vi "Test Broadcast Latest Message ID Correct.vi"(8 "error in (no error)":errorcluster, 11 "Test Case In":refnum<class "Debugger Test.lvclass">) -> (0 "error out":errorcluster, 3 "Test Case Out":refnum<class "Debugger Test.lvclass">)   [LabVIEW 2020, in "Debugger Test.lvclass"]
uses:
  Debugger Test.lvclass
  Debugger Test.lvclass/Debugger Test.ctl
  source/Process/Debug Process.lvclass
  source/Debugger/Debugger.lvclass
  source/Debug Data/Debug Data.lvclass
  source/Debug Data/Raw Debug Data.ctl
  C:/Users/anton/Documents/GitHub/triarc-debugger/source/Process/Debug Process.lvclass
  C:/Users/anton/Documents/GitHub/triarc-debugger/source/Debugger/Debugger.lvclass
  C:/Users/anton/Documents/GitHub/triarc-debugger/source/Debug Data Event/Debug Data Listener.lvclass
  25a4e40d-e468-46ca-96f8-86723b982b85.vi
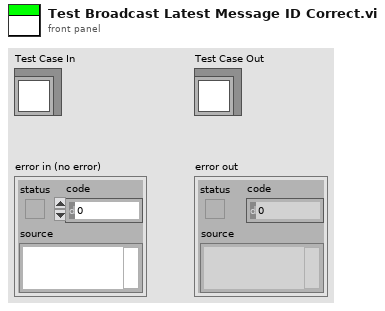
[diagram p1: front panel]
types:
  T1 = typedef "Debug Data.lvclass/Raw Debug Data.ctl" = cluster{"Action":string, "Call Chain":string, "Process":string, "Message":string, "Message Data":variant, "Time":dbl}
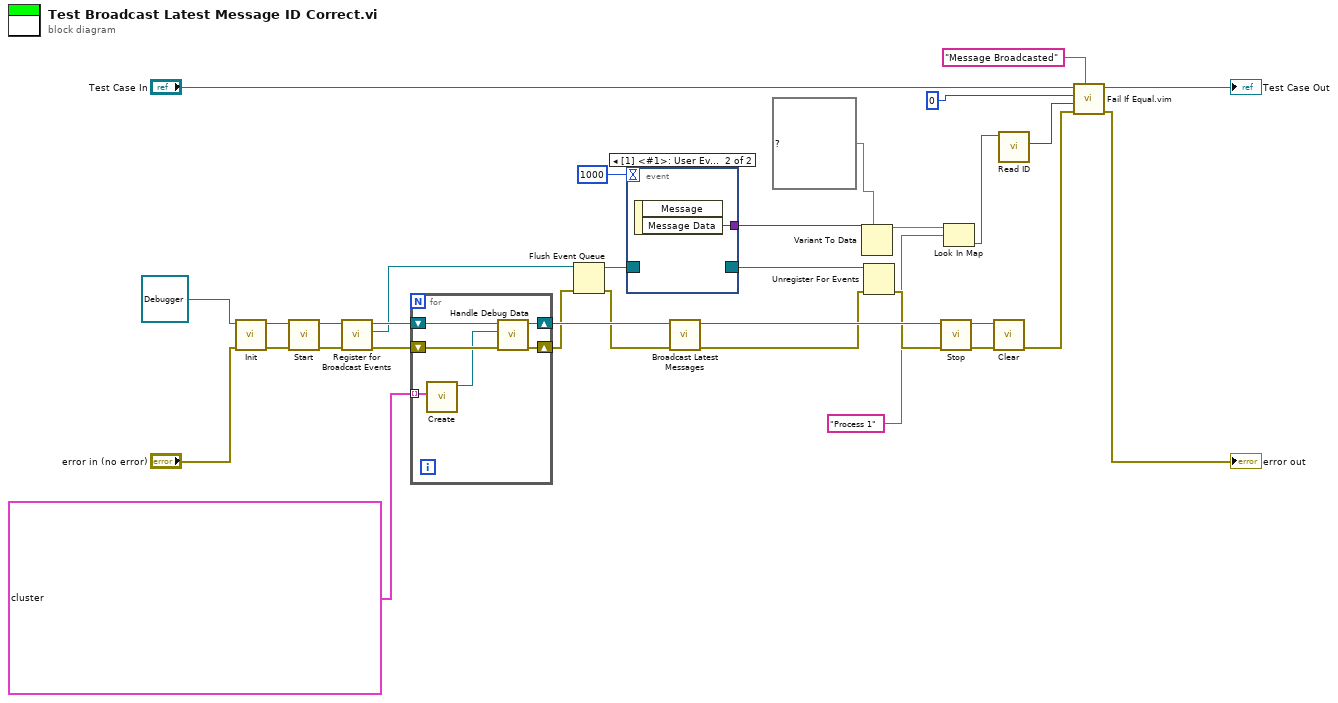
[diagram p0: block diagram]
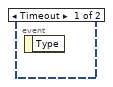
[diagram p2: hidden frame]
diagram:
  n1 = call-dynamic "Init.vi"("error in (no error)"="error in (no error)", "Process In"=refnum<class "Debugger.lvclass"> refnum ("Debug Data Event In 2")) -> ("error out"=w29:errorcluster, "Process Out"=w30:refnum<class "Debugger.lvclass">)  [unwired: 8 in]
  n2 = call "Start.vi"("error in (no error)"=w29, "Process In"=w30) -> ("error out"=w27:errorcluster, "Process Out"=w28:refnum<class "Debugger.lvclass">)  [unwired: 7 in, 1 out]
  n3 = call "Register for Broadcast Events.vi"("error in (no error)"=w27, "Process In"=w28) -> ("error out"=w26:errorcluster, "Event Registration Refnum Out"=w12:refnum<event-registration>, "Process Out"=w20:refnum<class "Debugger.lvclass">)  [unwired: 7 in]
  n4 = for {
    shift-right: [w37] -> w24
    shift-left: w26 -> [w39]
    shift-right: [w38] -> w25
    shift-left: w20 -> [w36]
    tunnel: T1[] [{"Action"="Send", "Call Chain"="Test.vi:123456", "Process"="Process 1", "Message"="Init", "Message Data"=variant, "Time"=0.0}, {"Action"="Receive", "Call Chain"="TF.lvlib:Process.lvclass:Handle Messages.vi:1960001", "Process"="Process 1", "Message"="Init", "Message Data"=variant, "Time"=0.0}, {"Action"="Send", "Call Chain"="Test.vi", "Process"="Process 1", "Message"="Start", "Message Data"=variant, "Time"=0.0}] ("Debug Data Cluster") -> [w35] mode=indexing
    n5 = call "Create.vi"("Debug Data Cluster"=w35) -> ("Debug Data out"=w34:refnum<class "Debug Data.lvclass">)  [unwired: 9 in, 1 out]
    n6 = call-dynamic "Handle Debug Data.vi"("error in (no error)"=w39, "Debug Data.lvclass"=w34, "Debug Data Event In"=w36) -> ("error out"=w37:errorcluster, "Debug Data Event Out"=w38:refnum<class "Debugger.lvclass">)  [unwired: 7 in]
  }
  n7 = Flush Event Queue(0:w12, 3:w24) -> (8:w11:refnum<event-registration>, 11:w13:errorcluster)  [unwired: 4 in, 1 out]
  n8 = event shown="[1] <#1>: User Event" {
    selector: w11 -> [_ _]
    dyn-events: [_ _] -> w15
    timeout: 1000 -> [_ _]
    tunnel: [_ w40] -> w8
    event Timeout {
      n9 = event-data() -> ()  [unwired: 1 in, 1 out]
    }
    event User Event {
      n10 = event-data() -> ("Message Data"=w40:variant)  [unwired: 1 in, 1 out]
    }
  }
  n11 = call "Broadcast Latest Messages.vi"("error in (no error)"=w13, "Debugger in"=w25) -> ("error out"=w10:errorcluster, "Debugger out"=w23:refnum<class "Debugger.lvclass">)  [unwired: 8 in]
  n12 = Variant To Data(type=map{string, refnum<class "Debug Data.lvclass">} {} ("Latest Messages"), Variant=w8) -> (data=w6:map{string, refnum<class "Debug Data.lvclass">})  [unwired: 1 in, 1 out]
  n13 = Unregister For Events(event registration refnum=w15, error in=w10) -> (error out=w9:errorcluster)
  n14 = call "Stop.vi"("error in (no error)"=w9, "Process In"=w23) -> ("error out"=w21:errorcluster, "Process Out"=w22:refnum<class "Debugger.lvclass">)  [unwired: 7 in, 1 out]
  n15 = Look In Map(map=w6, key="Process 1") -> (value=w5:refnum<class "Debug Data.lvclass">)  [unwired: 1 in, 1 out]
  n16 = call-dynamic "Clear.vi"("error in (no error)"=w21, "Process In"=w22) -> ("error out"=w17:errorcluster)  [unwired: 9 in]
  n17 = call "Read ID.vi"("Debug Data in"=w5) -> ("ID"=w2:u32)  [unwired: 9 in, 1 out]
  n18 = call "Fail If Equal.vim"("Description"="Message Broadcasted", "error in (no error)"=w17, "Actual"=w2, "Expected"=u32 0 ("ID"), "LUnit Test Case In"="Test Case In") -> ("error out"=→"error out":errorcluster, "LUnit Test Case Out"=→"Test Case Out":refnum<class "Debugger Test.lvclass">)  [unwired: 5 in]
